vi "VXM_MotorPosition.vi"() -> (1 "Position String":string, 3 "Array":string[](array[string]))   [LabVIEW 2020]
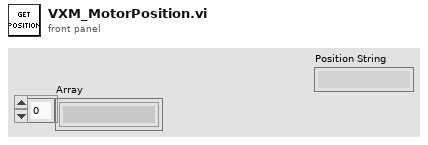
[diagram p1: front panel]
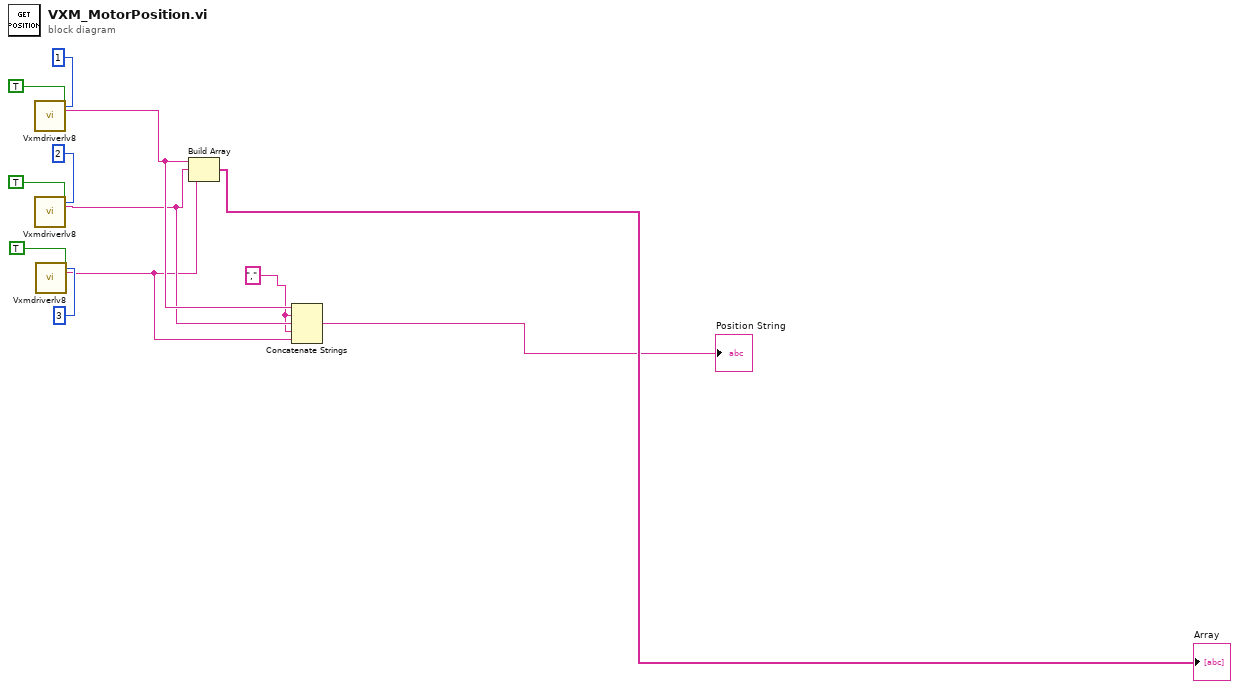
[diagram p0: block diagram]
diagram:
  w2 = "," ("string")
  n1 = call "Vxmdriverlv8.Vi"("Get\nMotor\nPosition"=TRUE ("Get\nMotor\nPosition"), "Motor\nNumber"=1 ("Motor\nNumber")) -> ("Motor Position"=w5:string)  [unwired: 20 in, 5 out]
  n2 = call "Vxmdriverlv8.Vi"("Get\nMotor\nPosition"=TRUE ("Get\nMotor\nPosition"), "Motor\nNumber"=2 ("Motor\nNumber")) -> ("Motor Position"=w4:string)  [unwired: 20 in, 5 out]
  n3 = call "Vxmdriverlv8.Vi"("Get\nMotor\nPosition"=TRUE ("Get\nMotor\nPosition"), "Motor\nNumber"=3 ("Motor\nNumber")) -> ("Motor Position"=w3:string)  [unwired: 20 in, 5 out]
  n4 = Build Array(w5, w4, w3) -> (→"Array":string[])
  n5 = Concatenate Strings(w5, w2, w4, w2, w3) -> (→"Position String":string)
